vi "SVN Checkout.vi"(8 "error in (no error)":errorcluster, 10 "ADT version":i32) -> (0 "error out":errorcluster, 1 "Successful Checkout":bool, 2 "Revision":i32, 3 "standard output":string, 4 "commandline":string)   [LabVIEW 2015, in "AguaClara Library.lvlib"]
uses:
  AguaClara Library.lvlib
  <vilib>/Utility/config.llb/NI_LVConfig.lvlib
  <vilib>/Utility/config.llb/Read Key (Boolean).vi
panel:
  out "standard error":string
  out "Ini file path":path
  out "Design Tool":path
  in  "Repository URL Final Designs":string="https://forge.cornell.edu/svn/repos/automated_design/Final Designs/"
  in  "command":string="cmd /c svn co"
  # "$ svn checkout -r 2 file:///var/svn/repos/test mine"
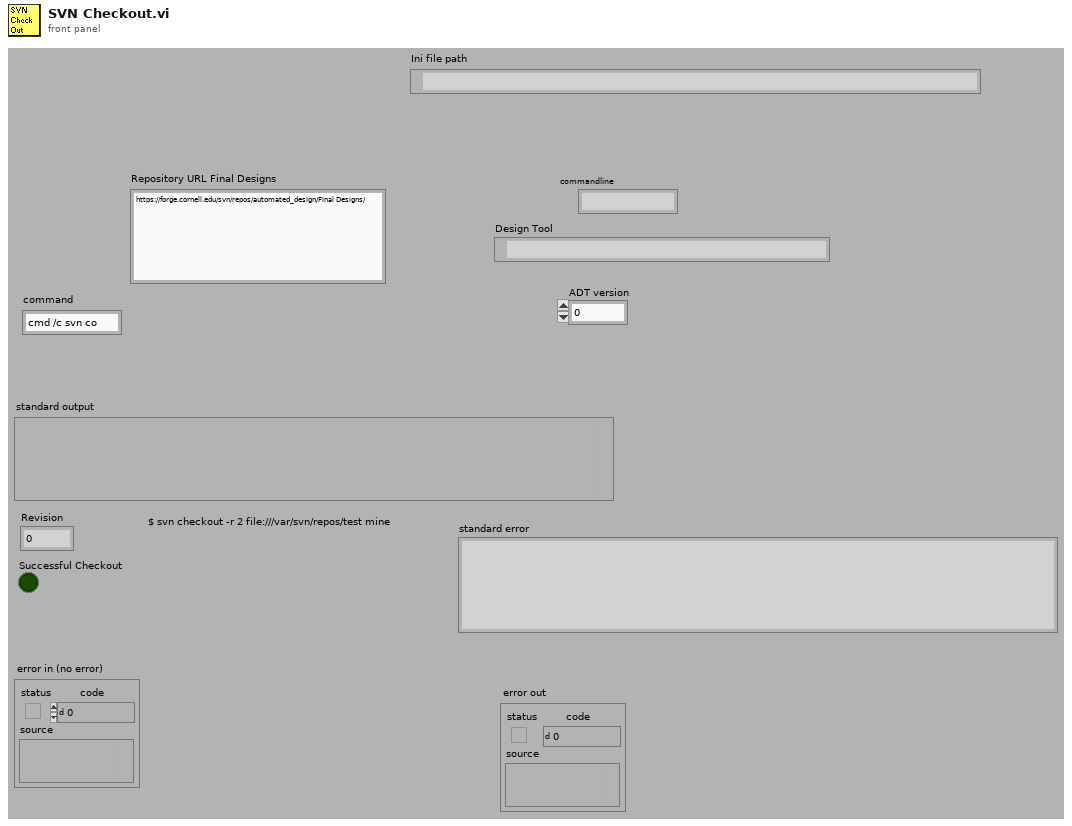
[diagram p1: front panel]
types:
  T1 = typedef "NI_LVConfig.lvlib/Config Data RefNum.ctl" = refnum<k1>
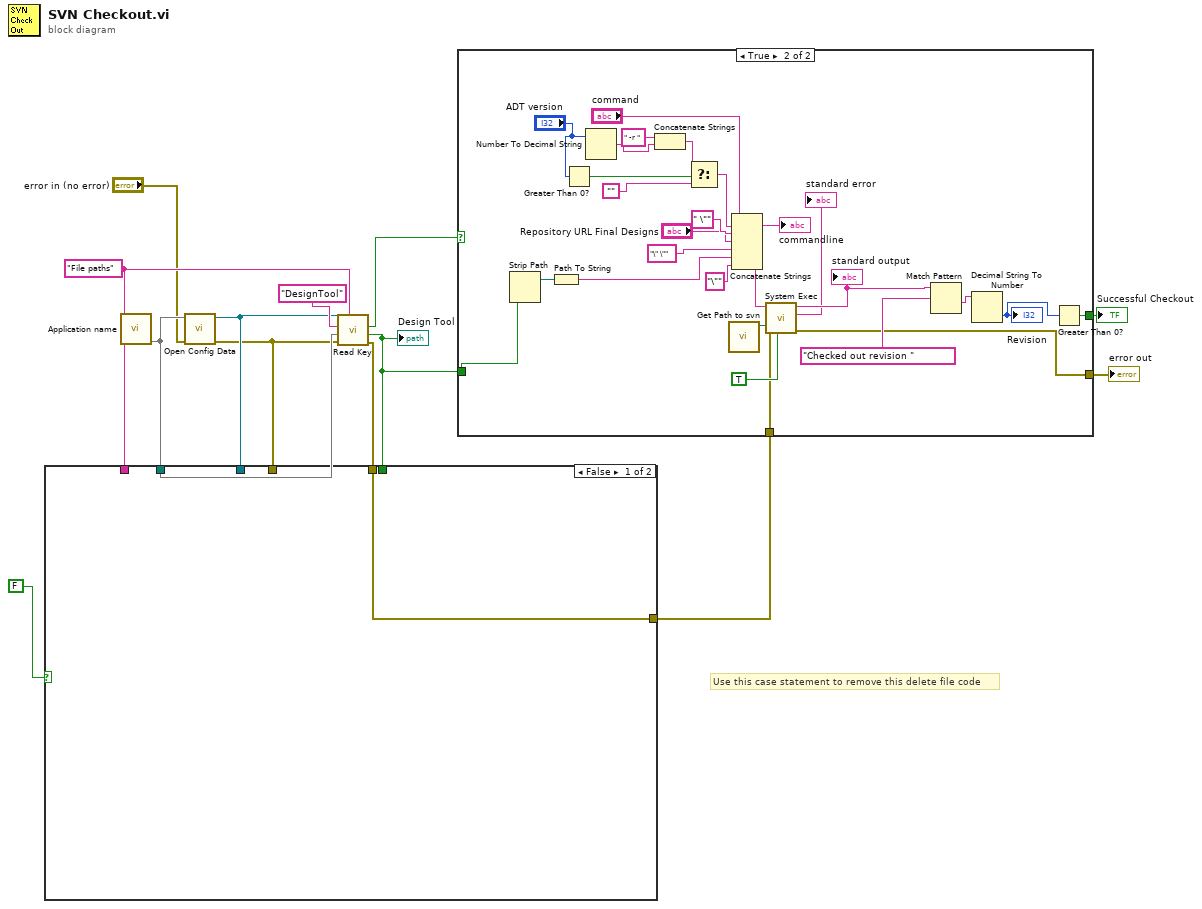
[diagram p0: block diagram]
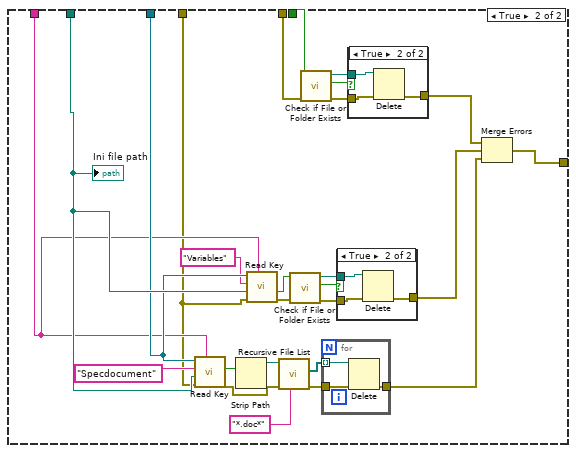
[diagram p3: hidden frame]
diagram:
  w9 = "File paths" ("section")
  # "Use this case statement to remove this delete file code"
  n1 = call "Application name.vi"() -> (0:w11)  [unwired: 4 in, 3 out]
  n2 = call <vilib>:"Open Config Data.vi"("error in (no error)"="error in (no error)", "configuration file path"=w11) -> ("error out"=w7:errorcluster, "refnum"=w10:T1)  [unwired: 7 in, 1 out]
  n3 = call-poly <vilib>:"Read Key.vi"("section"=w9, "error in (no error)"=w7, "default value"=w11, "key"="DesignTool", "refnum"=w10) -> ("error out"=w5:errorcluster, "value"=w6:bool, "found?"=w2:bool)  [unwired: 3 in, 1 out]
  "Design Tool" <- w6
  n4 = case shown="False" FALSE {
    tunnel: w11 -> [_ w38]
    tunnel: w10 -> [_ w37]
    tunnel: w9 -> [_ w35]
    tunnel: [w14 w33] -> w8
    tunnel: w7 -> [_ w32]
    tunnel: w6 -> [_ w26]
    tunnel: w5 -> [w14 w25]
    frame False {
    }
    frame True {
      n5 = call-poly <vilib>:"Read Key.vi"("section"=w35, "error in (no error)"=w32, "default value"=w38, "key"="Specdocument", "refnum"=w37) -> ("error out"=w30:errorcluster, "value"=w39:bool)  [unwired: 3 in, 2 out]
      n6 = Strip Path(path=w39) -> (stripped path=w31:path)  [unwired: 1 out]
      n7 = call-poly <vilib>:"Read Key.vi"("section"=w35, "error in (no error)"=w32, "default value"=w38, "key"="Variables", "refnum"=w37) -> ("error out"=w17:errorcluster, "value"=w18:bool)  [unwired: 3 in, 2 out]
      n8 = call <vilib>:"Recursive File List.vi"("pattern"="*.doc*", "error in (no error)"=w30, "Folder Path"=w31) -> ("error out"=w29:errorcluster, "All Files in Dir"=w28:path[])  [unwired: 4 in, 3 out]
      n9 = call <vilib>:"Check if File or Folder Exists.vi"("error in (no error)"=w17, "path"=w18) -> ("error out"=w19:errorcluster, "file or folder exists?"=w21:bool, "dup path"=w20:path)  [unwired: 7 in]
      n10 = call <vilib>:"Check if File or Folder Exists.vi"("error in (no error)"=w25, "path"=w26) -> ("error out"=w24:errorcluster, "file or folder exists?"=w22:bool, "dup path"=w23:path)  [unwired: 7 in]
      n11 = for {
        tunnel: w29 -> [w51]
        tunnel: w28 -> [w50] mode=indexing
        tunnel: [w49] -> w27
        n12 = Delete(path (use dialog)=w50, error in=w51) -> (error out=w49:errorcluster)  [unwired: 3 in, 2 out]
      }
      n13 = case shown="True" w21 {
        tunnel: [w41 w44] -> w16
        tunnel: w19 -> [w41 w43]
        tunnel: w20 -> [_ w42]
        frame False {
        }
        frame True {
          n14 = Delete(path (use dialog)=w42, error in=w43) -> (error out=w44:errorcluster)  [unwired: 3 in, 2 out]
        }
      }
      n15 = case shown="True" w22 {
        tunnel: [w45 w48] -> w34
        tunnel: w24 -> [w45 w47]
        tunnel: w23 -> [_ w46]
        frame False {
        }
        frame True {
          n16 = Delete(path (use dialog)=w46, error in=w47) -> (error out=w48:errorcluster)  [unwired: 3 in, 2 out]
        }
      }
      n17 = Merge Errors(w34, w16, w27) -> (w33:errorcluster)
      "Ini file path" <- w38
    }
  }
  n18 = case shown="True" w2 {
    selector: w2 -> [w53 _]
    tunnel: [w53 w68] -> w12
    tunnel: w8 -> [w52 w59]
    tunnel: w6 -> [_ w58]
    tunnel: [w52 w54] -> w1
    frame False {
    }
    frame True {
      n19 = Strip Path(path=w58) -> (stripped path=w78:path)  [unwired: 1 out]
      n20 = Path To String(path=w78) -> (string=w77:string)
      n21 = Greater Than 0?(x="ADT version") -> (x > 0?=w65:bool)
      n22 = Number To Decimal String(number="ADT version") -> (decimal integer string=w61:string)  [unwired: 1 in]
      n23 = Concatenate Strings(" -r " ("string"), w61) -> (w63:string)
      n24 = Select(t=w63, s=w65, f="") -> (s? t:f=w60:string)
      n25 = call "Get Path to svn.vi"() -> ("working directory"=w55:path)  [unwired: 7 in]
      n26 = Concatenate Strings("command", w60, " \"" ("string"), "Repository URL Final Designs", "\" \"" ("string"), w77, "\"" ("string")) -> (w76:string)
      "commandline" <- w76
      n27 = call <vilib>:"System Exec.vi"("run minimized? (F)"=TRUE, "error in (no error)"=w59, "working directory"=w55, "command line"=w76) -> ("error out"=w54:errorcluster, "standard error"=→"standard error":string, "standard output"=w72:string)  [unwired: 4 in, 1 out]
      "standard output" <- w72
      n28 = Match Pattern(string=w72, regular expression="Checked out revision ") -> (after substring=w70:string)  [unwired: 1 in, 3 out]
      n29 = Decimal String To Number(string=w70) -> (number=w69:i32)  [unwired: 2 in, 1 out]
      "Revision" <- w69
      n30 = Greater Than 0?(x=w69) -> (x > 0?=w68:bool)
    }
  }
  "Successful Checkout" <- w12
  "error out" <- w1
